vi "GetSubpanelPathsFromConfiguration.vi"(8 "error in (no error)":errorcluster, 10 "Path":path, 11 "SMO.UI.MAUI in":refnum<class "SMO.UI.MAUI.lvclass">) -> (0 "error out":errorcluster, 2 "Array":path[](array[path]), 3 "SMO.UI.MAUI out":refnum<class "SMO.UI.MAUI.lvclass">)   [LabVIEW 2020, in "SMO.UI.MAUI.lvclass"]
doc: "This VI will generate the specific locations for the subpanels. The subpanels for the different applications are stored as paths relative to the ini file they are stored in. This VI will build an array of paths from the array of relative paths located in the specific configuration file."
uses:
  SMO.UI.MAUI.lvclass
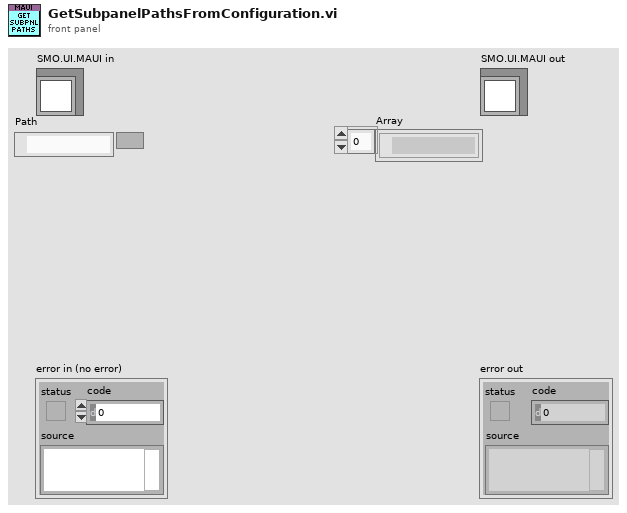
[diagram p1: front panel]
types:
  T1 = typedef "SMO.UI.MAUI.lvclass/SpecificConfiguration.ctl" = cluster{"Subpanels":string[]}
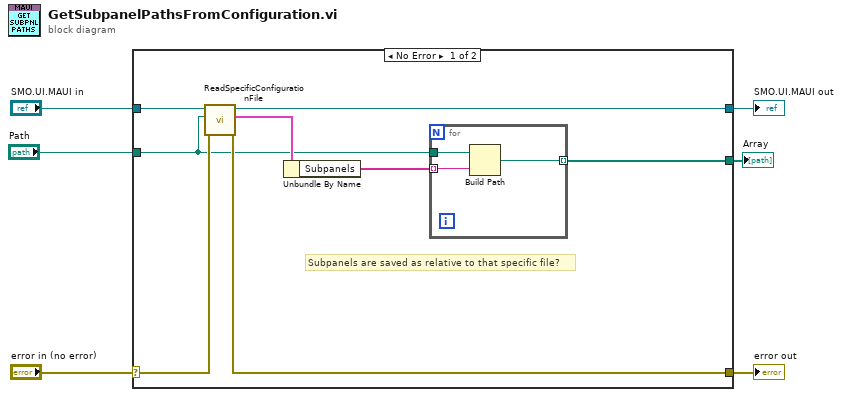
[diagram p0: block diagram]
diagram:
  n1 = case shown="No Error" "error in (no error)" {
    selector: "error in (no error)" -> [w12 w19]
    tunnel: [w11 w19] -> w5
    tunnel: [w14 w18] -> w3
    tunnel: "SMO.UI.MAUI in" -> [w13 w18]
    tunnel: "Path" -> [w8 _]
    tunnel: [w7 _] -> w1
    frame No Error {
      # "Subpanels are saved as relative to that specific file?"
      n2 = call "ReadSpecificConfigurationFile.vi"("error in (no error)"=w12, "Path"=w8, "SMO.UI.MAUI in"=w13) -> ("error out"=w11:errorcluster, "SpecificData"=w10:T1, "SMO.UI.MAUI out"=w14:refnum<class "SMO.UI.MAUI.lvclass">)  [unwired: 6 in]
      n3 = Unbundle By Name(w10) -> ("Subpanels"=w9:string[])
      n4 = for {
        tunnel: w9 -> [w17] mode=indexing
        tunnel: w8 -> [w16]
        tunnel: [w15] -> w7 mode=indexing
        n5 = Build Path(base path=w16, name or relative path=w17) -> (appended path=w15:path)
      }
    }
    frame Error {
    }
  }
  "error out" <- w5
  "SMO.UI.MAUI out" <- w3
  "Array" <- w1
